vi "ecg_ncs_v2c.vi"() -> ()   [LabVIEW 2016]
uses:
  <instrlib>/niUSRP/niUSRP Timestamp.ctl
  C:/Program Files/National Instruments/LabVIEW 2016/examples/Instrument IO/Serial/support/Serial - Settings.ctl
  <vilib>/Analysis/coordinate.llb/Wrap Angle (array).vi
  <vilib>/Instr/_visa.llb/VISA Configure Serial Port (Instr).vi
  <instrlib>/niUSRP/niUSRP Configure Time Start Trigger.vi
  <vilib>/Analysis/3filter.llb/Butterworth Filter (DBL).vi
  <instrlib>/niUSRP/niUSRP Write Tx Data (2D CDB).vi
  <instrlib>/niUSRP/niUSRP Fetch Rx Data (2D CDB).vi
  <vilib>/measure/NI_MABase.lvlib
  <vilib>/Analysis/NI_AALBase.lvlib
  <vilib>/Analysis/NI_AALPro.lvlib
  <vilib>/Analysis/NI_AAL_Angle.lvlib
panel:
  out "check counter":i32
  out "timed out?":bool
  out "#sample":i32=40819999
  in  "timeout in ms (-1)":i32=-1
  out "size(s) 3":i32=753
  out "size(s) 2":i32=1
  out "Serial Settings: \n#Bytes at Serial Port":u32=94
  in  "Stop":bool
  out "Poor Sensor Quality: \nSensor off":bool=TRUE
  out "Poor Sensor Quality: \nSensor on":bool
  out "Heart Rate 2":u16[](array[numeric])=[73]
  out "Stop Loop":bool=TRUE
  out "Loop index":i32=748
  out "size(s)":i32=753
  in  "Read Count":u32=80
  out "return count":u32=753
  in  "Serial Settings":T1={"baud rate"=57600, "data bits"=8, "parity"=enum."None", "stop bits"=10, "flow control"=0} {"flow control" items=["None"=0, "XON/XOFF"=1, "RTS/CTS"=2, "DTR/DSR"=4]; "stop bits" items=["1.0"=10, "1.5"=15, "2.0"=20]; "data bits" min=5 max=8 step=1; "baud rate" items=["75"=75, "110"=110, "134"=134, "150"=150, "300"=300, "600"=600, "1200"=1200, "1800"=1800, "2400"=2400, "4800"=4800, "7200"=7200, "9600"=9600, "14400"=14400, "19200"=19200, "28800"=28800, "38400"=38400, "56000"=56000, "57600"=57600, "115200"=115200, "128000"=128000, "230400"=230400]}
  in  "VISA resource name":refnum<visa-resource-name>="bmd101"
  in  "?":enum32{"ECG", "Heart Rate"}(tab)
  out "?":i16(graph)=131
  out "?":u8[](graph)=[73]
  in  "File Name":string="Test"
  in  "order1":i32=5
  in  "Path":path=path "D:/Research/SummerFall17Spring18/CnC/NCS/EcgNcsCorrelation"
  in  "Low-Pass Freq":dbl=200.0 format="%#_13g"
  in  "Sampling Rate":i32=500
  out "Gain":dbl=-15.0
  out "Bandwidth":dbl=56000000.0
  out "Coerced Carrier Frequency":dbl=2000000000.0 format="%#.17g"
  out "Coerced Tx IQ rate":dbl=1000000.0
  out "Coerced Rx IQ rate":dbl=1000000.0
  out "error IO":errorcluster={"status"=FALSE, "code"=-1074118647, "source"=""}
  in  "Rx Number of Samples":i32=20000
  in  "Tab Control 2":enum32{"NI-294x/295x", "NI-2900/2901"}(tab)=enum."NI-2900/2901"
  in  "channel 0 carrier\n frequency [Hz]":dbl=2000000000.0 format="%#_6p"
  in  "Rx carrier frequency [Hz]":dbl=2000000000.0 format="%#_6p"
  in  "Tx carrier frequency [Hz]":dbl=1000000000.0 format="%#_6p"
  in  "Start Trigger Time":T2={"whole seconds"=1, "fractional seconds"=0.0}
  out "Tx Active Antenna":string="TX1"
  in  "Tab Control":T3(tab)
  out "NCS tag Amp":dbl[](graph)=[1.823198297107392e-06]
  out "NCS tag Phase":dbl[](graph)=[0.03562971140940509]
  out "IQ":dbl[][](graph)=[[-0.008331551052877154], [0.0]]
  out "Tag Amp":dbl[](graph)=[0.008331551052877154]
  out "Tag Phase":dbl[](graph)=[337.4998459209021]
  out "Tx Waveform Graph":waveform(dbl)[](graph)
  in  "Channel 0\nTone Amplitude":dbl=0.707 step=0.05 format="%#.6g"
  in  "Channel 0 \nTone Frequency":dbl=5000.0 format="%#_6p"
  in  "Waveform Size":dbl=2000.0
  in  "Rx Active Antenna":string="RX2"
  in  "Device Name":refnum<k15>="MyB200"
  in  "Tx Gain":dbl=28.0 format="%#_6f"
  in  "Tx IQ Rate":dbl=1000000.0 format="%#_6p"
  in  "Rx Gain":dbl=32.0 format="%#_6f"
  in  "Rx IQ Rate":dbl=1000000.0 format="%#_6p"
  # "Rx Settings"
  # "Tx Settings"
  # "Note that on the NI-2900 and NI-2901, both Rx channels share an LO and both Tx channels share an LO. However, on the NI-294x/295x devices, Rx and Tx of channel 0 share an LO and Rx and Tx of channel 1 share an LO."
  # "This Tx graph should always have end and start tied up since this is being sent in a loop continuously. Otherwise phase jumps will be noticed."
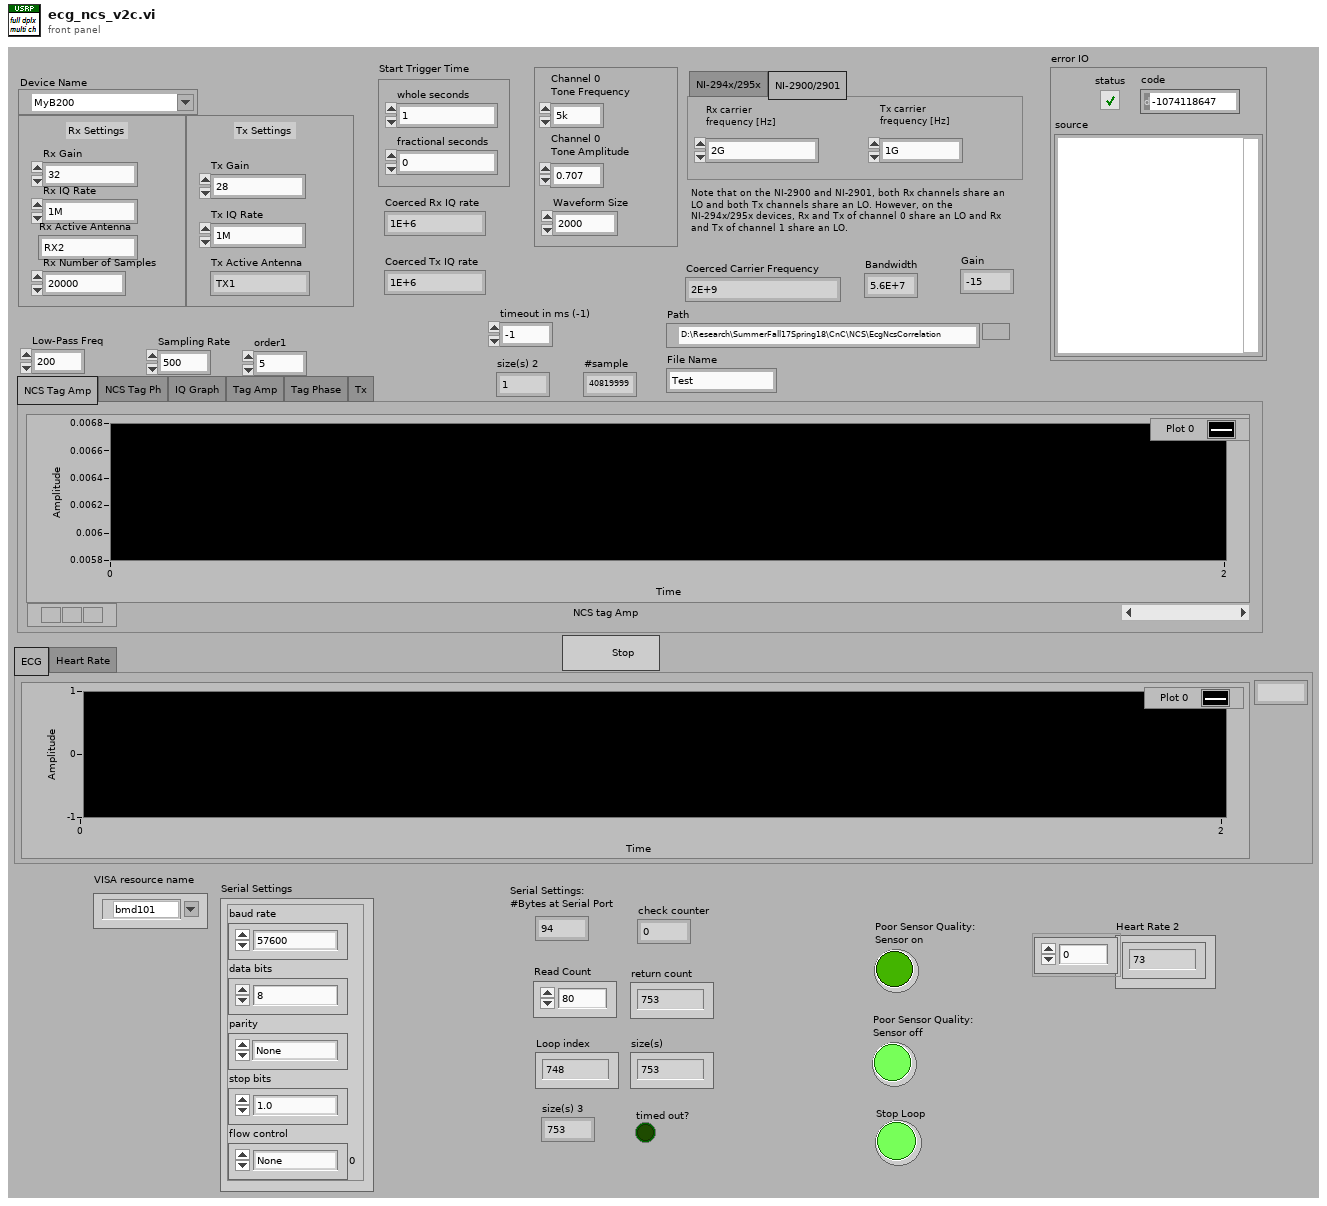
[diagram p1: front panel]
types:
  T1 = typedef "Serial - Settings.ctl" = cluster{"baud rate":u32, "data bits":u16, "parity":enum16{"None", "Odd", "Even", "Mark", "Space"}, "stop bits":u16, "flow control":u16}
  T2 = typedef "niUSRP Timestamp.ctl" = cluster{"whole seconds":u64, "fractional seconds":dbl}
  T3 = enum32{"NCS Tag Amp", "NCS Tag Ph", "IQ Graph", "Tag Amp", "Tag Phase", "Tx"}
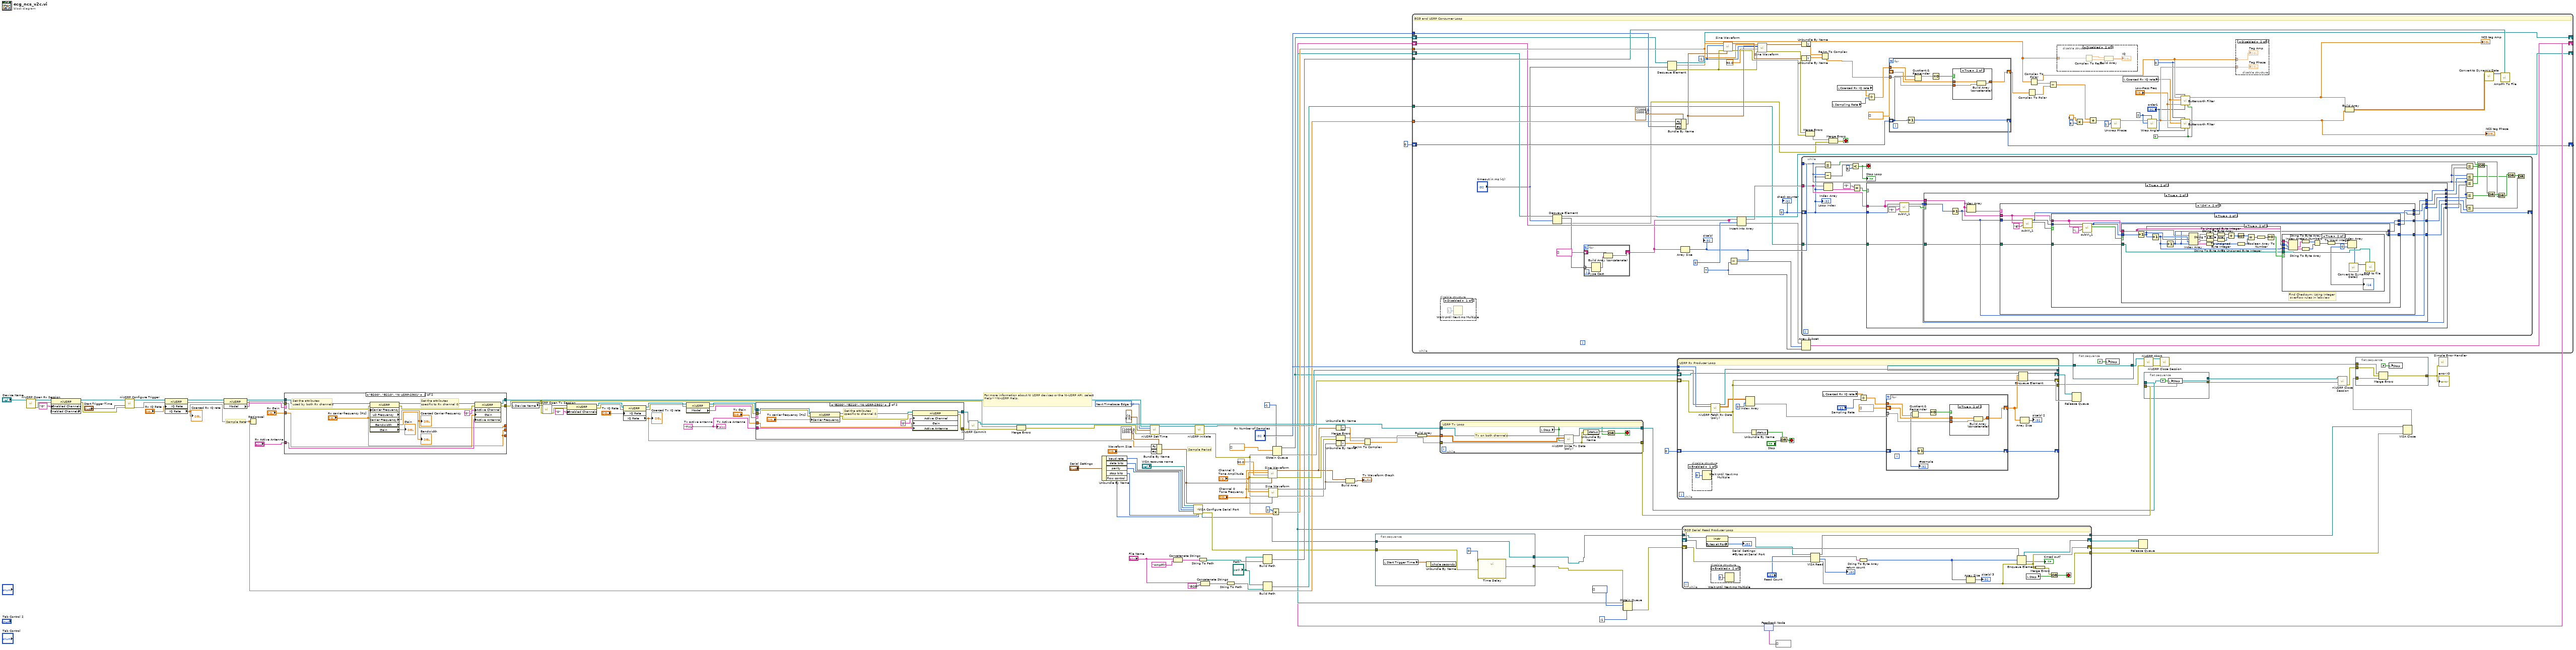
[diagram p0: block diagram]
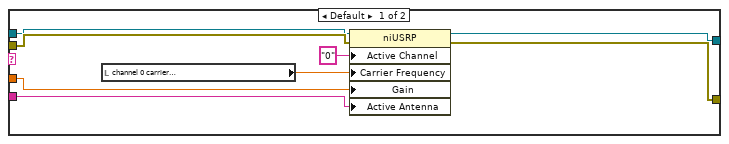
[diagram p5: hidden frame]
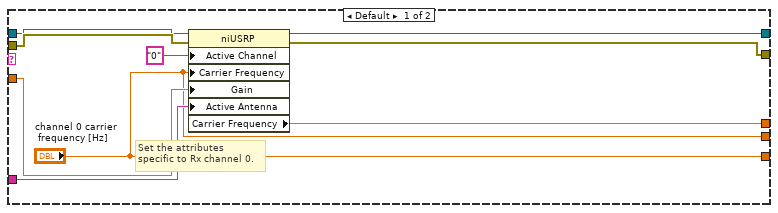
[diagram p6: hidden frame]
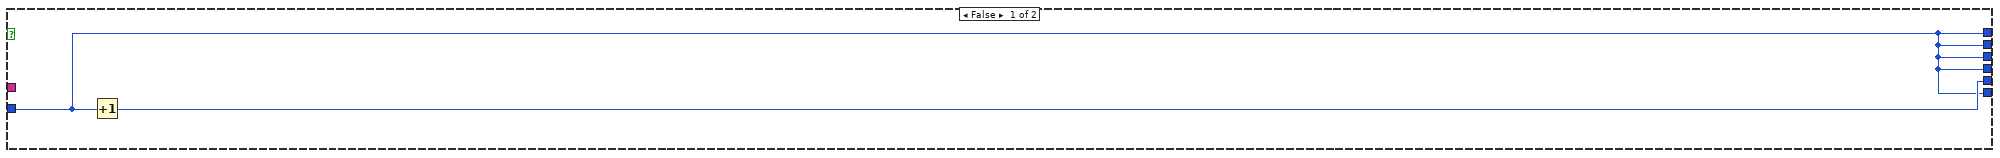
[diagram p9: hidden frame]
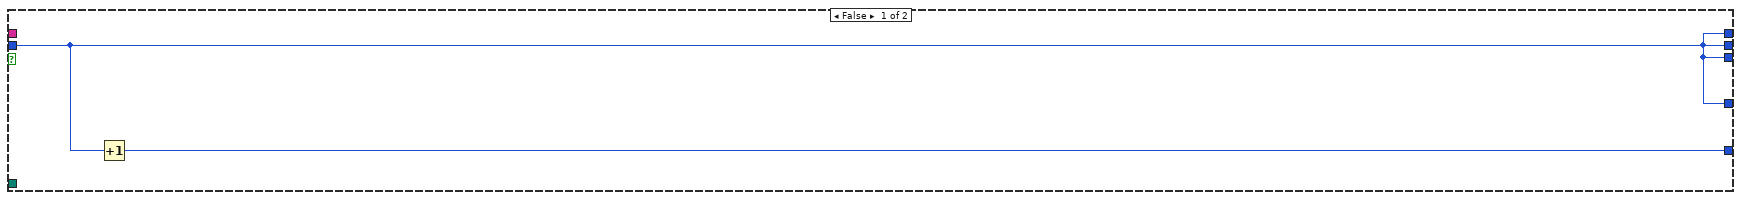
[diagram p10: hidden frame]
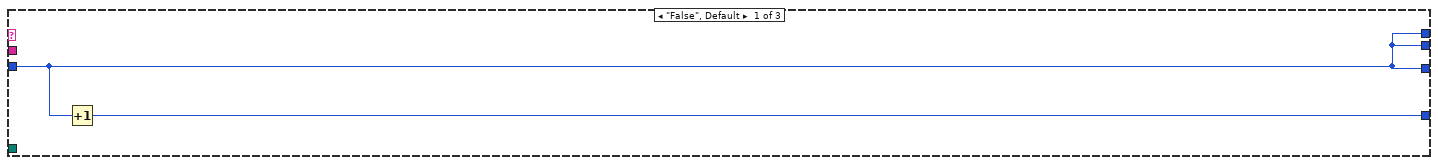
[diagram p11: hidden frame]
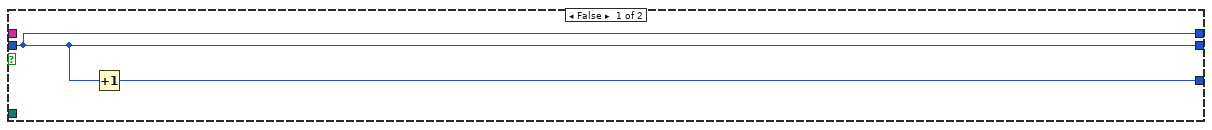
[diagram p12: hidden frame]
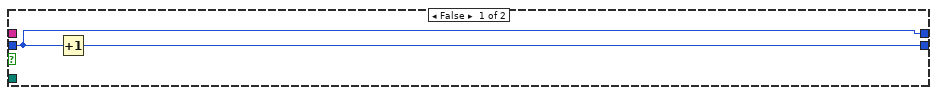
[diagram p13: hidden frame]
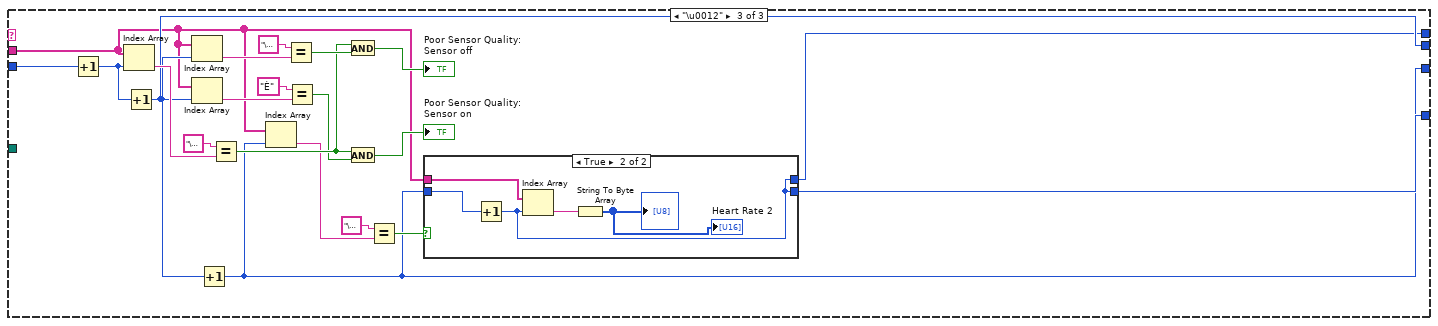
[diagram p15: hidden frame]
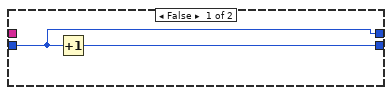
[diagram p16: hidden frame]
diagram:
  w93 = 1 items=["Now", "Next Timebase Edge"] ("apply timestamp")
  w62 = "TX1"  # Tx active antenna
  # "Sample Rate"
  # "Sample Period"
  # "For more information about NI USRP devices or the NI-USRP API, select Help>>NI-USRP Help."
  n1 = call <instrlib>:"niUSRP Open Rx Session.vi"("device names"="Device Name") -> ("session handle out"=w92:refnum<k15>, "error out"=w91:errorcluster)  [unwired: 13 in]
  n2 = property class="niUSRP" props=["Enabled Channels", "Enabled Channels"](reference=w92, error in=w91, "Enabled Channels"="0" ("Configuration:Enabled Channels")) -> (reference out=w90:refnum<k15>, error out=w89:errorcluster)  [unwired: 1 out]
  n3 = call-poly <instrlib>:"niUSRP Configure Trigger.vi"("session handle"=w90, "start trigger time"="Start Trigger Time", "error in (no error)"=w89) -> ("session handle out"=w86:refnum<k15>, "error out"=w85:errorcluster)  [unwired: 11 in]
  n4 = property class="niUSRP"(reference=w86, error in=w85, "IQ Rate"="Rx IQ Rate") -> (reference out=w82:refnum<k15>, error out=w83:errorcluster, "IQ Rate"=w21:dbl)
  "Coerced Rx IQ rate" <- w21
  n5 = property class="niUSRP"(reference=w82, error in=w83) -> (reference out=w77:refnum<k15>, error out=w78:errorcluster, "Model"=w79:string)
  n6 = Reciprocal(x=w21) -> ()  [unwired: 1 out]
  n7 = case shown="\"B200\", \"B210\", \"NI USRP-2901\"" w79 {
    tunnel: w78 -> [w126 w136]
    tunnel: w77 -> [w125 w137]
    tunnel: [w122 w133] -> w81
    tunnel: [w121 w132] -> w80
    tunnel: "Rx Gain" -> [w124 w139]
    tunnel: "Rx Active Antenna" -> [w123 w138]
    tunnel: [w119 w128] -> _
    tunnel: ["channel 0 carrier\n frequency [Hz]" "Rx carrier frequency [Hz]"] -> _
    tunnel: ["channel 0 carrier\n frequency [Hz]" "Rx carrier frequency [Hz]"] -> _
    frame Default {
      # "Set the attributes \nspecific to Rx channel 0."
      n8 = property class="niUSRP"(reference=w125, error in=w126, "Active Channel"="0", "Carrier Frequency"="channel 0 carrier\n frequency [Hz]", "Gain"=w124, "Active Antenna"=w123) -> (reference out=w122:refnum<k15>, error out=w121:errorcluster, "Carrier Frequency"=w119:dbl)
    }
    frame "B200", "B210", "NI USRP-2901" {
      # "Set the attributes \nused by both Rx channels"
      # "Set the attributes \nspecific to Rx channel 0."
      n9 = property class="niUSRP" props=["Carrier Frequency", "LO Frequency", "Carrier Frequency", "Bandwidth", "Gain"](reference=w137, error in=w136, "Carrier Frequency"="Rx carrier frequency [Hz]") -> (reference out=w135:refnum<k15>, error out=w134:errorcluster, "Carrier Frequency"=w128:dbl, "Bandwidth"=→"Bandwidth":dbl, "Gain"=→"Gain":dbl)  [unwired: 1 out]
      "Coerced Carrier Frequency" <- w128
      n10 = property class="niUSRP"(reference=w135, error in=w134, "Active Channel"="0", "Gain"=w139, "Active Antenna"=w138) -> (reference out=w133:refnum<k15>, error out=w132:errorcluster)
    }
  }
  n11 = local read "Device Name"() -> (w113:refnum<k15>)
  n12 = call <instrlib>:"niUSRP Open Tx Session.vi"("device names"=w113, "error in (no error)"=w80) -> ("session handle out"=w88:refnum<k15>, "error out"=w87:errorcluster)  [unwired: 12 in]
  n13 = property class="niUSRP"(reference=w88, error in=w87, "Enabled Channels"="0" ("Configuration:Enabled Channels")) -> (reference out=w74:refnum<k15>, error out=w73:errorcluster)
  n14 = property class="niUSRP"(reference=w74, error in=w73, "IQ Rate"="Tx IQ Rate") -> (reference out=w68:refnum<k15>, error out=w69:errorcluster, "IQ Rate"=w66:dbl)
  "Coerced Tx IQ rate" <- w66
  n15 = property class="niUSRP"(reference=w68, error in=w69) -> (reference out=w70:refnum<k15>, error out=w71:errorcluster, "Model"=w67:string)
  n16 = case shown="\"B200\", \"B210\", \"NI USRP-2901\"" w67 {
    tunnel: "Tx Gain" -> [w148 w158]
    tunnel: w62 -> [w146 w156]
    tunnel: [w142 w150] -> w64
    tunnel: [w141 w149] -> w65
    tunnel: w71 -> [w145 w152]
    tunnel: w70 -> [w144 w155]
    frame Default {
      n17 = local read "channel 0 carrier\n frequency [Hz]"() -> (w143:dbl)
      n18 = property class="niUSRP"(reference=w144, error in=w145, "Active Channel"="0", "Carrier Frequency"=w143, "Gain"=w148, "Active Antenna"=w146) -> (reference out=w142:refnum<k15>, error out=w141:errorcluster)
    }
    frame "B200", "B210", "NI USRP-2901" {
      # "Set the attributes \nspecific to channel 0."
      n19 = property class="niUSRP"(reference=w155, error in=w152, "Carrier Frequency"="Tx carrier frequency [Hz]") -> (reference out=w154:refnum<k15>, error out=w153:errorcluster)
      n20 = property class="niUSRP"(reference=w154, error in=w153, "Active Channel"="0", "Gain"=w158, "Active Antenna"=w156) -> (reference out=w150:refnum<k15>, error out=w149:errorcluster)
    }
  }
  n21 = call <instrlib>:"niUSRP Commit.vi"("session handle"=w64, "error in (no error)"=w65) -> ("session handle out"=w115:refnum<k15>, "error out"=w116:errorcluster)  [unwired: 12 in]
  n22 = Merge Errors(w80, w116) -> (w95:errorcluster)
  n23 = Unbundle By Name("Serial Settings") -> ("baud rate"=w28:u32, "data bits"=w29:u16, "parity"=w30:enum16{"None", "Odd", "Even", "Mark", "Space"}, "stop bits"=w31:u16, "flow control"=w32:u16)
  n24 = call <instrlib>:"niUSRP Set Time.vi"("session handle"=w81, "apply timestamp"=w93, "timestamp"=T2 {"whole seconds"=0, "fractional seconds"=0.0}, "error in (no error)"=w95) -> ("session handle out"=w97:refnum<k15>, "error out"=w96:errorcluster)  [unwired: 10 in]
  n25 = Bundle By Name(cluster=cluster{"Fs":dbl, "#s":dbl} {"Fs"=1000.0, "#s"=1000.0} ("sampling info"), "Fs"=w66, "#s"="Waveform Size") -> (w99:cluster{"Fs":dbl, "#s":dbl})
  n26 = Concatenate Strings("File Name", "AmpPh") -> (w46:string)
  n27 = call-poly "VISA Configure Serial Port"("VISA resource name"="VISA resource name", "baud rate (9600)"=w28, "data bits (8)"=w29, "parity (0:none)"=w30, "stop bits (10: 1 bit)"=w31, "flow control (0:none)"=w32) -> ("VISA resource name out"=w7:refnum<visa-resource-name>, "error out"=w8:errorcluster)  [unwired: 4 in, 4 out]
  n28 = call <instrlib>:"niUSRP Initiate.vi"("session handle"=w97, "error in (no error)"=w96) -> ("session handle out"=w24:refnum<k15>, "error out"=w11:errorcluster)  [unwired: 12 in]
  n29 = String To Path(string=w46) -> (path=w45:path)
  n30 = Concatenate Strings("File Name", "ECG") -> (w40:string)
  n31 = String To Path(string=w40) -> (path=w39:path)
  n32 = Build Path(base path="Path", name or relative path=w45) -> (appended path=w48:path)
  n33 = Build Path(base path="Path", name or relative path=w39) -> (appended path=w14:path)
  n34 = call <vilib>:"Sine Waveform.vi"("sampling info"=w99, "error in (no error)"=w11, "phase"=90.0, "amplitude"="Channel 0\nTone Amplitude", "frequency"="Channel 0 \nTone Frequency") -> ("error out"=w60:errorcluster, "signal out"=w107:waveform(dbl))  [unwired: 5 in]
  n35 = call <vilib>:"Sine Waveform.vi"("sampling info"=w99, "error in (no error)"=w11, "amplitude"="Channel 0\nTone Amplitude", "frequency"="Channel 0 \nTone Frequency") -> ("error out"=w61:errorcluster, "signal out"=w108:waveform(dbl))  [unwired: 6 in]
  n36 = Multiply(x=2, y="Channel 0 \nTone Frequency") -> (x*y=w49:dbl)
  n37 = Obtain Queue(max queue size (-1, unlimited)=-1, element data type=dbl[] [], error in (no error)=w11) -> (queue out=w16:refnum<queue>, error out=w20:errorcluster)  [unwired: 2 in, 1 out]
  n38 = Unbundle By Name(w107) -> ("Y"=w106:dbl[])
  n39 = Merge Errors(w60, w61) -> (w59:errorcluster)
  n40 = Unbundle By Name(w108) -> ("Y"=w105:dbl[])
  n41 = Build Array(w107, w108) -> (→"Tx Waveform Graph":waveform(dbl)[])
  n42 = Re/Im To Complex(1:w105, 2:w106) -> (0:w101:cdb[])
  n43 = flat-sequence {
    tunnel: w8 -> [w163]
    tunnel: [w162] -> w1
    tunnel: w7 -> [w161]
    tunnel: [w161] -> w2
    frame #0 {
      n44 = local read "Start Trigger Time"() -> (w160:T2)
      n45 = Unbundle By Name(w160) -> ()  [unwired: 1 out]
      n46 = call "Time Delay"("error in (no error)"=w163, "Delay Time (s)"=0) -> ("error out"=w162:errorcluster)  [unwired: 9 in]
    }
  }
  n47 = Build Array(w101) -> (w100:cdb[][])
  n48 = while {
    tunnel: w115 -> [w171]
    tunnel: w59 -> [w170]
    tunnel: [w168] -> w58
    tunnel: [w166] -> w54
    tunnel: w100 -> [w165]
    stop <- w167 stop-if-true
    # "Tx on both channels"
    # "USRP Tx Loop"
    n49 = local read "Stop"() -> (w164:bool)
    n50 = call-poly <instrlib>:"niUSRP Write Tx Data (poly).vi"("session handle"=w171, "data"=w165, "end of data?"=w164, "error in (no error)"=w170) -> ("session handle out"=w166:refnum<k15>, "error out"=w168:errorcluster)  [unwired: 10 in]
    n51 = Unbundle By Name(w168) -> ("status"=w169:bool)
    n52 = Compound Arithmetic op=OR(w169, w164) -> (w167:bool)
  }
  n53 = Obtain Queue(max queue size (-1, unlimited)=-1, element data type=i32[] [], error in (no error)=w1) -> (queue out=w13:refnum<queue>, error out=w34:errorcluster)  [unwired: 2 in, 1 out]
  n54 = while {
    tunnel: w24 -> [w192]
    tunnel: [w191] -> w23
    tunnel: "Rx Number of Samples" -> [w190]
    tunnel: [w184] -> w15
    shift-right: [w187] -> w18
    shift-left: w16 -> [w188]
    shift-right: [w186] -> w17
    shift-left: w20 -> [w185]
    shift-right: [w172] -> _
    shift-left: 0 -> [w173]
    stop <- w189 stop-if-true
    # "USRP Rx Producer Loop"
    n55 = disable-structure shown="Enabled" {
      frame Enabled {
        n56 = Wait Until Next ms Multiple(millisecond multiple=u32 0 ("milliseconds to wait")) -> ()  [unwired: 1 out]
      }
      frame Disabled {
      }
    }
    n57 = call-poly <instrlib>:"niUSRP Fetch Rx Data (poly).vi"("session handle"=w192, "number of samples"=w190, "error in (no error)"=w185) -> ("session handle out"=w191:refnum<k15>, "data"=w182:cdb[][], "error out"=w184:errorcluster)  [unwired: 9 in, 1 out]
    n58 = Index Array(array=w182, index (row)=0 ("y")) -> (element=w176:cdb[])  [unwired: 1 in]
    n59 = Unbundle By Name(w184) -> ("status"=w193:bool)
    n60 = Or(x=w193, y="Stop") -> (x .or. y?=w189:bool)
    n61 = local read "Coerced Rx IQ rate"() -> (w180:dbl)
    n62 = Divide(x=w180, y="Sampling Rate") -> (x/y=w178:dbl)
    n63 = for {
      tunnel: w176 -> [w201] mode=indexing
      shift-right: [w199] -> w175
      shift-left: dbl[] [] -> [w200]
      tunnel: w178 -> [w196]
      shift-right: [w194] -> w172
      shift-left: w173 -> [w195]
      n64 = Quotient & Remainder(x=w195, y=w196) -> (x-y*floor(x/y)=w197:dbl)  [unwired: 1 out]
      n65 = Increment(x=w195) -> (x+1=w194:i32)
      n66 = Equal To 0?(x=w197) -> (x = 0?=w198:bool)
      n67 = case shown="True" w198 {
        tunnel: w201 -> [_ w205]
        tunnel: w200 -> [w202 w204]
        tunnel: [w202 w203] -> w199
        frame False {
        }
        frame True {
          n68 = Build Array (concatenate)(w204, w205) -> (w203:cdb[])
        }
      }
      "#sample" <- w195
    }
    n69 = Enqueue Element(queue=w188, element=w175, error in (no error)=w184) -> (queue out=w187:refnum<queue>, error out=w186:errorcluster)  [unwired: 1 in, 1 out]
    n70 = Array Size(array=w175) -> (size(s)=→"size(s) 2":i32)
  }
  n71 = while {
    tunnel: [w215] -> w38
    shift-right: [w219] -> w36
    shift-left: w34 -> [w216]
    shift-right: [w220] -> w35
    shift-left: w13 -> [w221]
    tunnel: w2 -> [w214]
    tunnel: [w222] -> w37
    stop <- w224 stop-if-true
    # "ECG Serial Read Producer Loop"
    n72 = property class="Instr"(reference=w214) -> (reference out=w213:refnum<visa-resource-name>, "Bytes at Port"=→"Serial Settings: \n#Bytes at Serial Port":u32)  [unwired: 1 in, 1 out]
    n73 = disable-structure shown="Enabled" {
      frame Disabled {
      }
      frame Enabled {
        n74 = Wait Until Next ms Multiple(millisecond multiple=u32 0) -> ()  [unwired: 1 out]
      }
    }
    n75 = VISA Read(VISA resource name=w213, byte count="Read Count", error in (no error)=w216) -> (VISA resource name out=w222:refnum<visa-resource-name>, read buffer=w212:string, return count=→"return count":u32, error out=w215:errorcluster)
    n76 = String To Byte Array(string=w212) -> (unsigned byte array=w207:u8[])
    n77 = Array Size(array=w207) -> (size(s)=→"size(s) 3":i32)
    n78 = Enqueue Element(queue=w221, element=w207, error in (no error)=w215) -> (queue out=w220:refnum<queue>, timed out?=→"timed out?":bool, error out=w219:errorcluster)  [unwired: 1 in]
    n79 = local read "Stop"() -> (w217:bool)
    n80 = Merge Errors(w219) -> (w218:errorcluster)
    n81 = Or(x=w218, y=w217) -> (x .or. y?=w224:bool)
  }
  n82 = feedback #1(string[] []) -> (w6:string[])
  n83 = while {
    tunnel: "Rx Number of Samples" -> [w288]
    tunnel: w21 -> [w280]
    tunnel: w49 -> [w281]
    tunnel: w48 -> [w279]
    shift-right: [w257] -> _
    shift-left: w16 -> [w258]
    tunnel: w14 -> [w236]
    shift-right: [w249] -> _
    shift-left: w13 -> [w250]
    shift-right: [w247] -> w12
    shift-left: w6 -> [w246]
    shift-right: [w231] -> _
    shift-left: 0 -> [w232]
    stop <- w248 stop-if-true
    w254 = 7
    w251 = 0
    w268 = 2 ("y")
    w261 = TRUE
    w263 = 0
    w286 = -1
    # "ECG and USRP Consumer Loop"
    n84 = disable-structure shown="Disabled" {
      frame Disabled {
        n85 = Wait Until Next ms Multiple(millisecond multiple=u32 1) -> ()  [unwired: 1 out]
      }
      frame Enabled {
      }
    }
    n86 = Dequeue Element(queue=w250, timeout in ms (-1)="timeout in ms (-1)") -> (queue out=w249:refnum<queue>, element=w228:i32[], error out=w226:errorcluster)  [unwired: 1 in, 1 out]
    n87 = for {
      tunnel: w228 -> [w294] mode=indexing
      shift-right: [w291] -> w227
      shift-left: string[] [] -> [w292]
      n88 = Type Cast(x=w294) -> (*(type *) &x=w293:string)  [unwired: 1 in]
      n89 = Build Array (concatenate)(w292, w293) -> (w291:string[])
    }
    n90 = Dequeue Element(queue=w258, timeout in ms (-1)="timeout in ms (-1)") -> (queue out=w257:refnum<queue>, element=w243:dbl[], error out=w245:errorcluster)  [unwired: 1 in, 1 out]
    n91 = Bundle By Name(cluster=cluster{"Fs":dbl, "#s":dbl} {"Fs"=1000.0, "#s"=1000.0} ("sampling info"), "Fs"=w280, "#s"=w288) -> (w285:cluster{"Fs":dbl, "#s":dbl})
    n92 = Array Size(array=w227) -> (size(s)=w252:i32)
    "size(s)" <- w252
    n93 = call <vilib>:"Sine Waveform.vi"("sampling info"=w285, "error in (no error)"=w245, "amplitude"=w286, "frequency"=w281) -> ("error out"=w284:errorcluster, "signal out"=w289:waveform(dbl))  [unwired: 6 in]
    n94 = Subtract(x=w252, y=w254) -> (x-y=w253:i32)
    n95 = Insert Into Array(array=w227, index=0, new element=w246) -> (w255:string[])
    n96 = call <vilib>:"Sine Waveform.vi"("sampling info"=w285, "error in (no error)"=w245, "phase"=90.0, "amplitude"=w286, "frequency"=w281) -> ("error out"=w283:errorcluster, "signal out"=w282:waveform(dbl))  [unwired: 5 in]
    n97 = Unbundle By Name(w282) -> ("Y"=w277:dbl[])
    n98 = Unbundle By Name(w289) -> ("Y"=w276:dbl[])
    n99 = while {
      tunnel: w255 -> [w329]
      shift-right: [w333] -> _
      shift-left: w251 -> [w312]
      tunnel: w252 -> [w313]
      tunnel: w236 -> [w308]
      stop <- w309 stop-if-true
      n100 = Less Or Equal?(x=w313, y=w312) -> (x <= y?=w314:bool)
      n101 = Subtract(x=w313, y=w312) -> (x-y=w311:i32)
      n102 = Index Array(array=w329, index=w312) -> (element=w332:string)
      n103 = Less?(x=w311, y=6) -> (x < y?=w309:bool)
      "Stop Loop" <- w309
      n104 = Equal?(x="ª", y=w332) -> (x = y?=w330:bool)
      n105 = case shown="True" w330 {
        tunnel: w312 -> [w334 w345]
        tunnel: [w335 w343] -> w333
        tunnel: w329 -> [_ w337]
        tunnel: [w334 w342] -> w328
        tunnel: [w334 w341] -> w326
        tunnel: [w334 w340] -> w323
        tunnel: [w334 w339] -> w320
        tunnel: [w334 w338] -> w317
        tunnel: w308 -> [_ w336]
        frame False {
          n106 = Increment(x=w334) -> (x+1=w335:i32)
        }
        frame True {
          n107 = call "subVI_1.vi"("String"="ª", "Array"=w337, "Numeric in"=w345) -> ("Boolean"=w344:bool, "Numeric out"=w342:i32)  [unwired: 7 in]
          n108 = case shown="True" w344 {
            tunnel: w342 -> [w347 w351]
            tunnel: [w348 w357] -> w343
            tunnel: w337 -> [_ w356]
            tunnel: [w347 w352] -> w341
            tunnel: [w347 w355] -> w340
            tunnel: [w347 w354] -> w339
            tunnel: [w347 w353] -> w338
            tunnel: w336 -> [_ w349]
            frame False {
              n109 = Increment(x=w347) -> (x+1=w348:i32)
            }
            frame True {
              n110 = Increment(x=w351) -> (x+1=w352:i32)
              n111 = Index Array(array=w356, index=w352) -> (element=w350:string)
              n112 = case shown="\"\\04\"" w350 {
                tunnel: w352 -> [w358 w365 w433]
                tunnel: [w359 w368 w415] -> w357
                tunnel: w356 -> [_ w361 w417]
                tunnel: [w358 w363 w419] -> w355
                tunnel: [w358 w367 w416] -> w354
                tunnel: [w358 w366 w414] -> w353
                tunnel: w349 -> [_ w360 _]
                frame "False", Default {
                  n113 = Increment(x=w358) -> (x+1=w359:i32)
                }
                frame "\u0004" {
                  n114 = call "subVI_1.vi"("String"="€", "Array"=w361, "Numeric in"=w365) -> ("Boolean"=w362:bool, "Numeric out"=w363:i32)  [unwired: 7 in]
                  n115 = case shown="True" w362 {
                    tunnel: w363 -> [w369 w376]
                    tunnel: [w370 w378] -> w368
                    tunnel: w361 -> [_ w375]
                    tunnel: [w369 w373] -> w367
                    tunnel: [w369 w377] -> w366
                    tunnel: w360 -> [_ w371]
                    frame False {
                      n116 = Increment(x=w369) -> (x+1=w370:i32)
                    }
                    frame True {
                      n117 = call "subVI_1.vi"("String"="\u0002", "Array"=w375, "Numeric in"=w376) -> ("Boolean"=w372:bool, "Numeric out"=w373:i32)  [unwired: 7 in]
                      n118 = case shown="True" w372 {
                        tunnel: w373 -> [w379 w385]
                        tunnel: [w380 w382] -> w378
                        tunnel: w375 -> [_ w386]
                        tunnel: [w379 w382] -> w377
                        tunnel: w371 -> [_ w381]
                        frame False {
                          n119 = Increment(x=w379) -> (x+1=w380:i32)
                        }
                        frame True {
                          # "Find Checksum: Using Integer\n overflow rules in labview"
                          n120 = Increment(x=w385) -> (x+1=w384:i32)
                          n121 = Increment(x=w384) -> (x+1=w383:i32)
                          n122 = Increment(x=w383) -> (x+1=w382:i32)
                          n123 = Index Array(array=w386, index #1=w384, index #2=w383, index #3=w382) -> (element #1=w400:string, element #2=w399:string, element #3=w393:string)
                          n124 = String To Byte Array(string=w400) -> (unsigned byte array=w398:u8[])
                          n125 = String To Byte Array(string=w399) -> (unsigned byte array=w397:u8[])
                          n126 = String To Byte Array(string=w393) -> (unsigned byte array=w392:u8[])
                          n127 = To Unsigned Byte Integer(number=w398) -> (unsigned 8bit integer=w396:u8[])
                          n128 = To Unsigned Byte Integer(number=w397) -> (unsigned 8bit integer=w395:u8[])
                          n129 = Add(x=w396, y=w395) -> (x+y=w394:u8[])
                          n130 = Not(x=w394) -> (.not. x?=w391:u8[])
                          n131 = To Unsigned Byte Integer(number=w392) -> (unsigned 8bit integer=w390:u8[])
                          n132 = Equal?(x=w391, y=w390) -> (x = y?=w389:bool[])
                          n133 = Boolean Array To Number(Boolean array=w389) -> (number=w388:u32)
                          n134 = Equal To 0?(x=w388) -> (x = 0?=w387:bool)
                          n135 = case shown="True" w387 {
                            tunnel: w386 -> [_ w413]
                            tunnel: w384 -> [_ w407]
                            tunnel: w383 -> [_ w406]
                            tunnel: w381 -> [_ w403]
                            frame False {
                            }
                            frame True {
                              n136 = Index Array(array=w413, index #1=w407, index #2=w406) -> (element #1=w412:string, element #2=w411:string)
                              n137 = String To Byte Array(string=w412) -> (unsigned byte array=w410:u8[])
                              n138 = String To Byte Array(string=w411) -> (unsigned byte array=w409:u8[])
                              n139 = Join Numbers(hi=w410, lo=w409) -> ((hi.lo)=w408:u16[])
                              n140 = To Word Integer(number=w408) -> (16bit integer=w405:i16[])
                              n141 = Index Array(array=w405, index=0) -> (element=w402:i16)
                              "?" <- w402
                              n142 = call "Convert to Dynamic Data2"("Double"=w402) -> ("Dynamic Data Type"=w401:dynamicdata)  [unwired: 3 in]
                              n143 = call "ECG to file"("Signals"=w401, "Filename"=w403) -> ()  [unwired: 15 in, 3 out]
                            }
                          }
                        }
                      }
                    }
                  }
                }
                frame "\u0012" {
                  n144 = Increment(x=w433) -> (x+1=w429:i32)
                  n145 = Index Array(array=w417, index=w429) -> (element=w432:string)
                  n146 = Increment(x=w429) -> (x+1=w419:i32)
                  n147 = Index Array(array=w417, index=w419) -> (element=w430:string)
                  n148 = Index Array(array=w417, index=w419) -> (element=w427:string)
                  n149 = Increment(x=w419) -> (x+1=w414:i32)
                  n150 = Equal?(x="\u0002", y=w432) -> (x = y?=w424:bool)
                  n151 = Index Array(array=w417, index=w414) -> (element=w420:string)
                  n152 = Equal?(x="\u0000", y=w430) -> (x = y?=w426:bool)
                  n153 = Equal?(x="È", y=w427) -> (x = y?=w423:bool)
                  n154 = And(x=w424, y=w426) -> (x .and. y?=→"Poor Sensor Quality: \nSensor off":bool)
                  n155 = And(x=w424, y=w423) -> (x .and. y?=→"Poor Sensor Quality: \nSensor on":bool)
                  n156 = Equal?(x="\u0003", y=w420) -> (x = y?=w418:bool)
                  n157 = case shown="True" w418 {
                    tunnel: w414 -> [w435 w441]
                    tunnel: w417 -> [_ w440]
                    tunnel: [w435 w439] -> w416
                    tunnel: [w436 w439] -> w415
                    frame False {
                      n158 = Increment(x=w435) -> (x+1=w436:i32)
                    }
                    frame True {
                      n159 = Increment(x=w441) -> (x+1=w439:i32)
                      n160 = Index Array(array=w440, index=w439) -> (element=w438:string)
                      n161 = String To Byte Array(string=w438) -> (unsigned byte array=→"Heart Rate 2" →"?":u8[])
                    }
                  }
                }
              }
            }
          }
        }
      }
      n162 = Less Or Equal?(x=w313, y=w323) -> (x <= y?=w321:bool)
      n163 = Less Or Equal?(x=w313, y=w320) -> (x <= y?=w318:bool)
      n164 = Less Or Equal?(x=w313, y=w328) -> (x <= y?=w327:bool)
      n165 = Less Or Equal?(x=w313, y=w326) -> (x <= y?=w324:bool)
      n166 = Less Or Equal?(x=w313, y=w317) -> (x <= y?=w315:bool)
      n167 = Or(x=w314, y=w327) -> (x .or. y?=w325:bool)
      n168 = Or(x=w325, y=w324) -> (x .or. y?=w322:bool)
      n169 = Or(x=w322, y=w321) -> (x .or. y?=w319:bool)
      n170 = Or(x=w319, y=w318) -> (x .or. y?=w316:bool)
      n171 = Or(x=w316, y=w315) -> ()  [unwired: 1 out]
      "Loop index" <- w312
    }
    n172 = Array Subset(array=w227, index=w253, length=w254) -> (w247:string[])
    n173 = Merge Errors(w283, w284) -> (w244:errorcluster)
    n174 = Re/Im To Complex(1:w276, 2:w277) -> (0:w239:cdb[])
    n175 = Merge Errors(w244, w226) -> (w248:errorcluster)
    n176 = local read "Sampling Rate"() -> (w237:i32)
    n177 = local read "Coerced Rx IQ rate"() -> (w241:dbl)
    n178 = Divide(x=w241, y=w237) -> (x/y=w240:dbl)
    n179 = for {
      tunnel: w239 -> [w303] mode=indexing
      shift-right: [w301] -> w238
      shift-left: dbl[] [] -> [w302]
      tunnel: w240 -> [w298]
      shift-right: [w296] -> w231
      shift-left: w232 -> [w297]
      n180 = Increment(x=w297) -> (x+1=w296:i32)
      n181 = Quotient & Remainder(x=w297, y=w298) -> (x-y*floor(x/y)=w299:dbl)  [unwired: 1 out]
      n182 = Equal To 0?(x=w299) -> (x = 0?=w300:bool)
      n183 = case shown="True" w300 {
        tunnel: w303 -> [_ w307]
        tunnel: w302 -> [w304 w306]
        tunnel: [w304 w305] -> w301
        frame False {
        }
        frame True {
          n184 = Build Array (concatenate)(w306, w307) -> (w305:cdb[])
        }
      }
    }
    n185 = Complex To Polar(r * e^(i*theta)=w238) -> (theta=w271:dbl[])  [unwired: 1 out]
    n186 = Complex To Polar(r * e^(i*theta)=w243) -> (r=w278:dbl[], theta=w266:dbl[])
    n187 = Subtract(x=w266, y=w271) -> (x-y=w270:dbl[])
    n188 = disable-structure shown="Disabled" {
      disable-tunnel: w243 -> [_ w444]
      frame Enabled {
      }
      frame Disabled {
        n189 = Complex To Re/Im(x + iy=w444) -> (x=w447:dbl[], y=w446:dbl[])
        n190 = Build Array(w447, w446) -> (→"IQ":dbl[][])
      }
    }
    n191 = Multiply(x=3.141592653589793, y=6) -> (x*y=w272:dbl)
    n192 = Add(x=w270, y=w272) -> (x+y=w269:dbl[])
    n193 = call <vilib>:"Unwrap Phase.vi"("phase unit"=1 ("y"), "Phase"=w269) -> ("Unwrapped Phase"=w267:dbl[])  [unwired: 8 in, 1 out]
    n194 = local read "Coerced Rx IQ rate"() -> (w264:dbl)
    n195 = call-poly <vilib>:"Wrap Angle.vi"("angle units"=w268, "angle range"=w268, "Angle In"=w267) -> ("Angle Out"=w265:dbl[])  [unwired: 7 in, 1 out]
    n196 = call-poly <vilib>:"Butterworth Filter.vi"("init/cont (init:F)"=w261, "order"="order1", "filter type"=w263, "low cutoff freq: fl"="Low-Pass Freq", "sampling freq: fs"=w264, "X"=w278) -> ("Filtered X"=w235:dbl[])  [unwired: 2 in, 1 out]
    "NCS tag Amp" <- w235
    n197 = call-poly <vilib>:"Butterworth Filter.vi"("init/cont (init:F)"=w261, "order"="order1", "filter type"=w263, "low cutoff freq: fl"="Low-Pass Freq", "sampling freq: fs"=w264, "X"=w265) -> ("Filtered X"=w234:dbl[])  [unwired: 2 in, 1 out]
    "NCS tag Phase" <- w234
    n198 = disable-structure shown="Disabled" {
      disable-tunnel: w278 -> [_ w443]
      disable-tunnel: w265 -> [_ w442]
      frame Enabled {
      }
      frame Disabled {
        "Tag Amp" <- w443
        "Tag Phase" <- w442
      }
    }
    n199 = Build Array(w235, w234) -> (w233:dbl[][])
    n200 = call "Convert to Dynamic Data"("2D Array"=w233) -> ("Dynamic Data Type"=w259:dynamicdata)  [unwired: 3 in]
    n201 = call "AmpPh To File"("Signals"=w259, "Filename"=w279) -> ()  [unwired: 15 in, 3 out]
    "check counter" <- w251
  }
  n202 = feedback-in #1(w12) -> ()
  n203 = Release Queue(queue=w18, error in (no error)=w17) -> ()  [unwired: 1 in, 3 out]
  n204 = flat-sequence {
    tunnel: [w448] -> w56
    tunnel: w23 -> [w448]
    frame #0 {
      n205 = local write "Stop"(TRUE ("STOP")) -> ()
    }
  }
  n206 = Release Queue(queue=w35, error in (no error)=w36) -> ()  [unwired: 1 in, 3 out]
  n207 = call <instrlib>:"niUSRP Abort.vi"("session handle"=w56, "error in (no error)"=w15) -> ("session handle out"=w112:refnum<k15>, "error out"=w111:errorcluster)  [unwired: 12 in]
  n208 = flat-sequence {
    tunnel: [w451] -> w57
    tunnel: w58 -> [w451]
    tunnel: [w450] -> w55
    tunnel: w54 -> [w450]
    frame #0 {
      n209 = local write "Stop"(TRUE ("STOP")) -> ()
    }
  }
  n210 = call <instrlib>:"niUSRP Close Session.vi"("session handle"=w112, "error in (no error)"=w111) -> ("error out"=w52:errorcluster)  [unwired: 13 in]
  n211 = call <instrlib>:"niUSRP Close Session.vi"("session handle"=w55, "error in (no error)"=w57) -> ("error out"=w53:errorcluster)  [unwired: 13 in]
  n212 = flat-sequence {
    tunnel: w53 -> [w456]
    tunnel: [w455] -> w44
    tunnel: w52 -> [w454]
    tunnel: w25 -> [w453]
    frame #0 {
      n213 = Merge Errors(w454, w456, w453) -> (w455:errorcluster)
      n214 = local write "Stop"(FALSE ("STOP")) -> ()
    }
  }
  n215 = VISA Close(VISA resource name=w37, error in (no error)=w38) -> (error out=w25:errorcluster)
  n216 = call <vilib>:"Simple Error Handler.vi"("error in (no error)"=w44) -> ()  [unwired: 1 in, 8 out]
  "Tx Active Antenna" <- w62
  "error IO" <- w44
